vi "Set TDF - Filter Impulse response.vi"(0 "reference in":refnum<class "GSwFormDSP.lvclass">, 5 "error in (no error)":errorcluster, 7 "Filter Impulse Response (TDF)":waveform(dbl)) -> (14 "reference out":refnum<class "GSwFormDSP.lvclass">, 19 "error out":errorcluster)   [LabVIEW 2022 SP3, in "GSwFormDSP.lvclass"]
uses:
  GSwFormDSP.lvclass
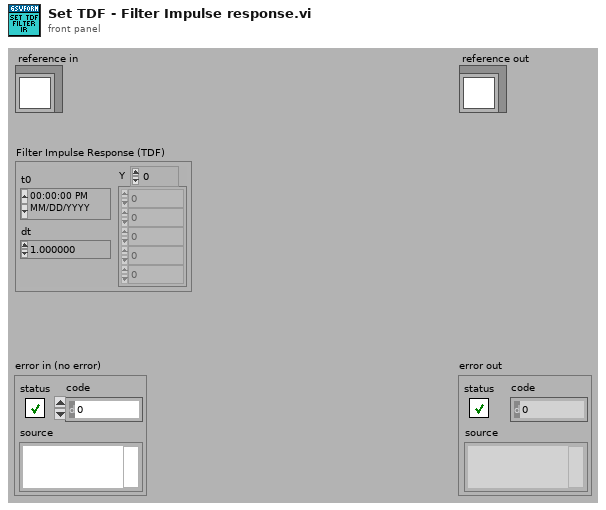
[diagram p1: front panel]
types:
  T1 = typedef "GSwFormDSP.lvclass/ObjectAttributesRef.ctl" = refnum<data-value>
  T2 = typedef "GSwFormDSP.lvclass/ObjectAttributes.ctl" = cluster{"Wform Ref":refnum<data-value>, "Nb Signals":i32, "Spectral Function Parameters":T3, "FFT":waveform(cdb)[], "Nb FFT":i32, "Nb Averages":i32[], "Reference Indexes":i32[], "Response Indexes":i32[], "Coherence":waveform(dbl)[], "TDF Parameters":T5, "DAQ":cluster{"Duration (sec)":dbl, "Buffer Size (Samples)":i32, "Offset (Samples)":i32}, "Filter Impulse Response (TDF)":waveform(dbl), "Sound Playback":T6}
  T3 = typedef "GSwFormDSP.lvclass/Spectral Parameters.ctl" = cluster{"Frequency resolution (Hz)":dbl, "Overlap":dbl, "Window":T4}
  T4 = typedef "NI_AALPro.lvlib/windowTd.ctl" = u32
  T5 = typedef "GSwFormDSP.lvclass/TDF Parameters.ctl" = cluster{"Filter":enum32{"Lowpass", "Highpass", "Bandpass", "Bandstop"}, "Type:":enum16{"Butterworth", "Chebyshev", "Inv Chebyshev", "Elliptic", "Bessel"}, "LP cutoff freq":dbl, "HP cutoff freq":dbl, "Order":i32, "passband ripple (dB)":dbl, "stopband attenuation (dB)":dbl, "Phaseless Filter":bool, "Include Fade IN and OUT":bool}
  T6 = typedef "GSwFormDSP.lvclass/Sound Playback.ctl" = cluster{"Timer start (ms)":u32, "task ID":T7, "Cursor Init Location (s)":dbl, "SC Volume":dbl}
  T7 = typedef "Sound Output Task ID.ctl" = u32
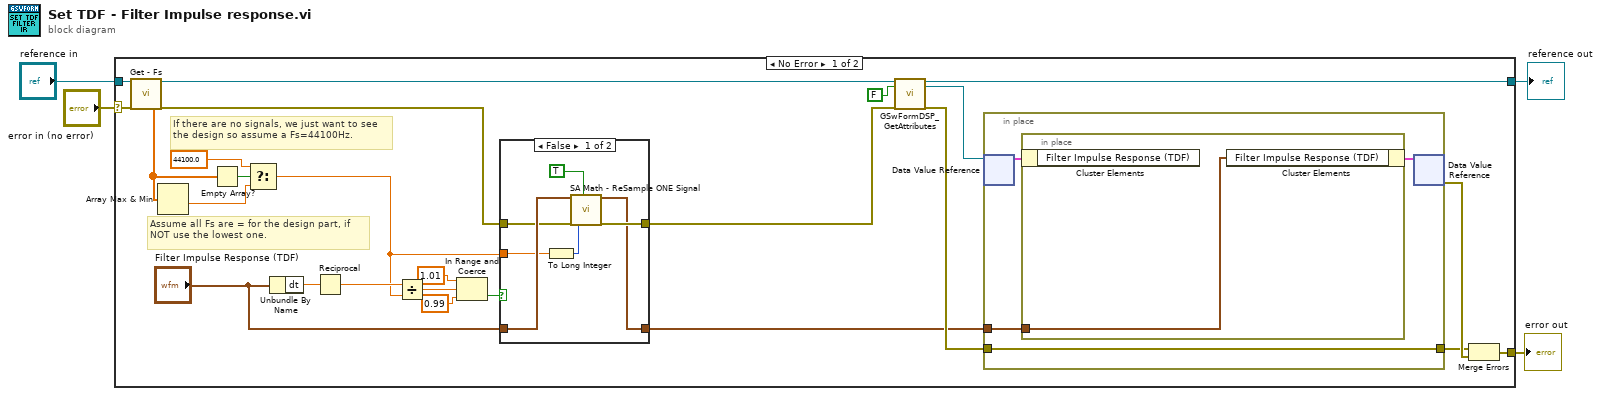
[diagram p0: block diagram]
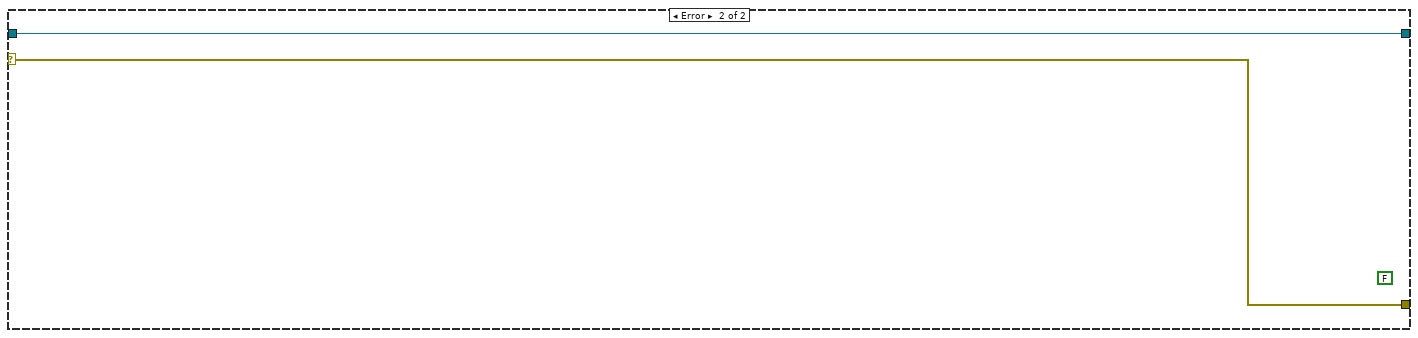
[diagram p3: hidden frame]
diagram:
  n1 = case shown="No Error" "error in (no error)" {
    selector: "error in (no error)" -> [w17 w45]
    tunnel: [w29 w45] -> w3
    tunnel: [w24 w44] -> w1
    tunnel: "reference in" -> [w18 w44]
    frame No Error {
      # "If there are no signals, we just want to see the design so assume a Fs=44100Hz."
      # "Assume all Fs are = for the design part, if NOT use the lowest one."
      n2 = call-dynamic "Get - Fs.vi"("reference in"=w18, "error in (no error)"=w17) -> ("Signals Fs"=w22:dbl[], "reference in"=w16:refnum<class "GSwFormDSP.lvclass">, "error out"=w7:errorcluster)  [unwired: 14 in, 1 out]
      n3 = Array Max & Min(array=w22) -> (min value=w20:dbl)  [unwired: 3 out]
      n4 = Empty Array?(array=w22) -> (empty?=w21:bool)
      n5 = Select(t=44100.0, s=w21, f=w20) -> (s? t:f=w5:dbl)
      n6 = Unbundle By Name("Filter Impulse Response (TDF)") -> ("dt"=w15:dbl)
      n7 = Reciprocal(x=w15) -> (1/x=w14:dbl)
      n8 = Divide(x=w14, y=w5) -> (x/y=w13:dbl)
      n9 = In Range and Coerce(upper limit=1.01, x=w13, lower limit=0.99 ("upper limit")) -> (In Range?=w10:bool)  [unwired: 1 out]
      n10 = case shown="False" w10 {
        tunnel: [w30 w38] -> w9
        tunnel: "Filter Impulse Response (TDF)" -> [w36 w38]
        tunnel: w7 -> [w35 w37]
        tunnel: [w34 w37] -> w6
        tunnel: w5 -> [w33 _]
        frame False {
          n11 = To Long Integer(number=w33) -> (32bit integer=w32:i32)
          n12 = call "SA Math - ReSample ONE Signal.vi"("wForm IN"=w36, "error in (no error)"=w35, "New Fs"=w32, "Anotate Signal Name"=TRUE) -> ("wForm OUT"=w30:waveform(dbl), "error out"=w34:errorcluster)  [unwired: 13 in, 1 out]
        }
        frame True {
        }
      }
      n13 = call "GSwFormDSP_GetAttributes.vi"("reference in"=w16, "return data? (T)"=FALSE, "error in (no error)"=w6) -> ("reference out"=w24:refnum<class "GSwFormDSP.lvclass">, "attributes ref"=w23:T1, "error out"=w25:errorcluster)  [unwired: 13 in, 1 out]
      n14 = in-place {
        in-place-border: w25 -> [w40]
        in-place-border: [w40] -> w27
        in-place-border: w9 -> [w39]
        n15 = in-place-dvr #1(w23) -> (w41:T2)  [unwired: 1 out]
        n16 = in-place {
          in-place-border: w39 -> [w43]
          n17 = in-place-cluster #2(w41) -> ()  [unwired: 1 out]
          n18 = in-place-cluster #2("Filter Impulse Response (TDF)"=w43) -> (w42:T2)
        }
        n19 = in-place-dvr #1(w42) -> (w28:errorcluster)  [unwired: 1 out]
      }
      n20 = Merge Errors(w27, w28) -> (w29:errorcluster)
    }
    frame Error {
      (unwired) FALSE
    }
  }
  "error out" <- w3
  "reference out" <- w1
